vi "Extract_line_data.vi"() -> ()   [LabVIEW 2020]
uses:
  <vilib>/Analysis/1siggen.llb/Ramp Pattern by Samples.vi
  <vilib>/Analysis/NI_AALBase.lvlib
panel:
  out "Profile":dbl[](graph)
  out "Intensity Graph":dbl[][](graph)
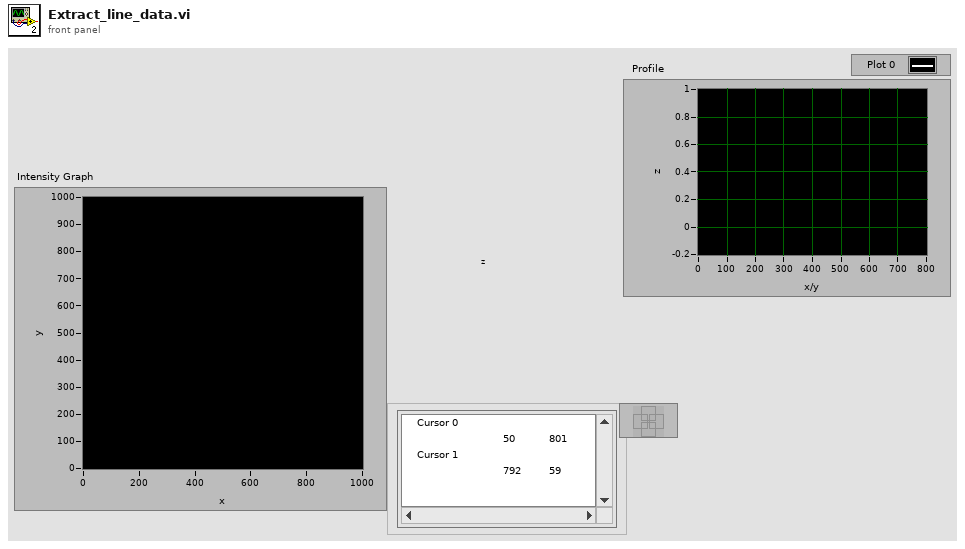
[diagram p1: front panel]
types:
  T1 = typedef "LVPointDoubleTypeDef.ctl" = cluster{"Cursor X":dbl, "Cursor Y":dbl}
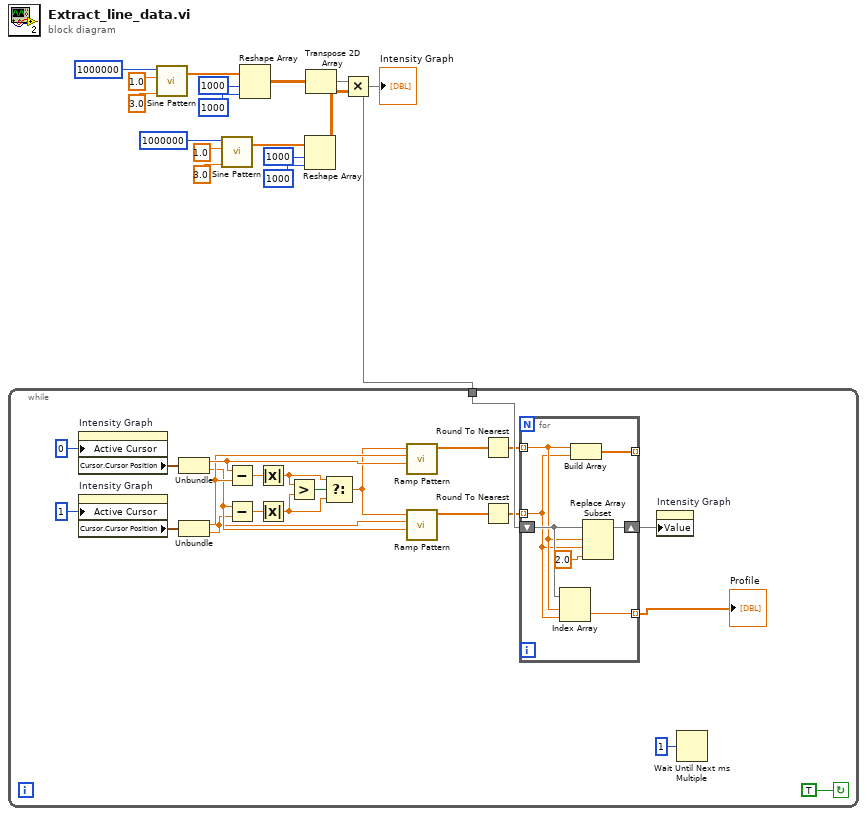
[diagram p0: block diagram]
diagram:
  n1 = call <vilib>:"Sine Pattern.vi"("cycles"=3.0, "amplitude"=1.0, "samples"=1000000) -> ("Sinusoidal Pattern"=w9:dbl[])  [unwired: 1 in, 1 out]
  n2 = call <vilib>:"Sine Pattern.vi"("cycles"=3.0, "amplitude"=1.0, "samples"=1000000) -> ("Sinusoidal Pattern"=w12:dbl[])  [unwired: 1 in, 1 out]
  n3 = Reshape Array(w9, 1000 ("dimension size"), 1000 ("dimension size")) -> (w4:dbl[][])
  n4 = Reshape Array(w12, 1000 ("dimension size"), 1000 ("dimension size")) -> (w3:dbl[][])
  n5 = Transpose 2D Array(2D array=w4) -> (transposed array=w2:dbl[][])
  n6 = Multiply(x=w2, y=w3) -> (x*y=w1:dbl[][])
  "Intensity Graph" <- w1
  n7 = while {
    tunnel: w1 -> [w39]
    stop <- TRUE continue-if-true
    n8 = property on="Intensity Graph" class="IntGraph (strict)"("Active Cursor"=u32 0) -> ("Cursor.Cursor Position"=w32:T1)  [unwired: 2 in, 2 out]
    n9 = property on="Intensity Graph" class="IntGraph (strict)"("Active Cursor"=u32 1) -> ("Cursor.Cursor Position"=w31:T1)  [unwired: 2 in, 2 out]
    n10 = Unbundle(w32) -> ("Cursor X"=w28:dbl, "Cursor Y"=w25:dbl)
    n11 = Unbundle(w31) -> ("Cursor X"=w27:dbl, "Cursor Y"=w23:dbl)
    n12 = Subtract(x=w28, y=w27) -> (x-y=w26:dbl)
    n13 = Subtract(x=w25, y=w23) -> (x-y=w24:dbl)
    n14 = Absolute Value(x=w26) -> (abs(x)=w21:dbl)
    n15 = Absolute Value(x=w24) -> (abs(x)=w20:dbl)
    n16 = Greater?(x=w21, y=w20) -> (0:w22:bool)
    n17 = Select(t=w21, s=w22, f=w20) -> (s? t:f=w19:dbl)
    n18 = call-poly <vilib>:"Ramp Pattern.vi"("start"=w28, "end"=w27, "samples"=w19) -> ("Ramp Pattern"=w38:dbl[])  [unwired: 7 in, 1 out]
    n19 = call-poly <vilib>:"Ramp Pattern.vi"("start"=w25, "end"=w23, "samples"=w19) -> ("Ramp Pattern"=w37:dbl[])  [unwired: 7 in, 1 out]
    n20 = Round To Nearest(number=w38) -> (nearest integer value=w36:dbl[])
    n21 = Round To Nearest(number=w37) -> (nearest integer value=w35:dbl[])
    n22 = for {
      shift-right: [w46] -> w18
      shift-left: w39 -> [w45]
      tunnel: w36 -> [w43] mode=indexing
      tunnel: w35 -> [w42] mode=indexing
      tunnel: [w41] -> _ mode=indexing
      tunnel: [w40] -> w17 mode=indexing
      n23 = Index Array(array=w45, index (row)=w43, index (col)=w42) -> (element=w40:dbl)
      n24 = Build Array(w43, w42) -> (w41:dbl[])
      n25 = Replace Array Subset(array=w45, new element=2.0 ("new element/subarray"), index (row)=w43, index (col)=w42) -> (w46:dbl[][])
    }
    "Profile" <- w17
    n26 = property on="Intensity Graph" class="IntGraph (strict)"("Value"=w18) -> ()  [unwired: 2 in, 2 out]
    n27 = Wait Until Next ms Multiple(millisecond multiple=u32 1) -> ()  [unwired: 1 out]
  }
